vi "Log Location.vi"() -> (2 "Log Location":path)   [LabVIEW 2020, in "RxnRover.lvlib" / "File IO.lvlib" / "Project Locations.lvlib"]
doc: "Returns the location of logs for the application, independent of whether it is run with the LabVIEW runtime, as a standalone EXE, using an installer, or during development in LabVIEW."
uses:
  Project Locations.lvlib
  AppData Utilities/LocalAppData Utilities.lvlib
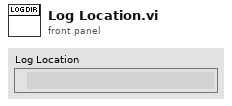
[diagram p1: front panel]
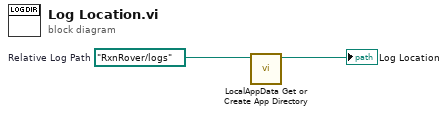
[diagram p0: block diagram]
diagram:
  w2 = path "RxnRover/logs"  # Relative Log Path
  n1 = call "LocalAppData Get or Create App Directory.vi"("Relative Path"=w2) -> ("Ouput File Path"=→"Log Location":path)  [unwired: 9 in, 1 out]
